vi "LV_MQTT_MDML_example.vi"() -> ()   [LabVIEW 2018]
uses:
  Downloads/mqtt_lv2013_201708181938/mqtt_lv2013/mqtt Folder/src/class/mqtt/mqttTypedef/mqttConnectionStatus.ctl
  Downloads/mqtt_lv2013_201708181938/mqtt_lv2013/mqtt Folder/src/class/mqtt/mqttTypedef/mqttConnectionMeta.ctl
  Downloads/mqtt_lv2013_201708181938/mqtt_lv2013/mqtt Folder/src/class/mqtt/mqttTypedef/mqttQOSlevel.ctl
  Downloads/mqtt_lv2013_201708181938/mqtt_lv2013/mqtt Folder/src/class/mqtt/mqttTypedef/mqttWillInformation.ctl
  vector_data.ctl
  query_part.ctl
  Downloads/mqtt_lv2013_201708181938/mqtt_lv2013/mqtt Folder/src/class/mqtt/mqtt.lvclass
panel:
  in  "Experiment ID 3":string
  in  "connMeta 7":T1
  in  "Device ID":string="DEVICE_A"
  in  "Experiment ID 2":string
  in  "Device ID":string
  in  "connMeta 6":T1
  in  "User Info":T3={"User Name"="test", "Password"="testtest"}
  in  "client":string
  in  "connMeta 5":T1
  in  "Experiment ID3":string
  in  "Configuration Filepath":path
  in  "Experiment ID":string
  in  "Experiment ID2":string
  in  "connMeta 4":T1
  out "error out 2":errorcluster
  in  "connMeta 3":T1
  out "sessionPresent":bool
  out "connStatus":T4
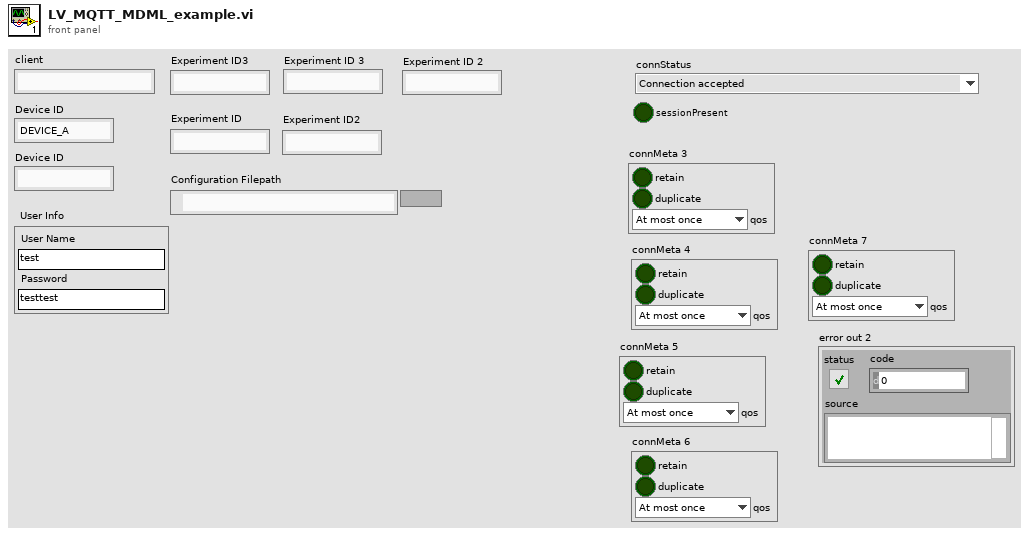
[diagram p1: front panel]
types:
  T1 = typedef "mqttConnectionMeta.ctl" = cluster{"retain":bool, "duplicate":bool, "qos":T2}
  T2 = typedef "mqttQOSlevel.ctl" = enum8{"At most once", "At least once", "Exactly once", "Reserved"}
  T3 = typedef "mqttWillInformation.ctl" = cluster{"User Name":string, "Password":string}
  T4 = typedef "mqttConnectionStatus.ctl" = enum16{"Connection accepted", "Connection refused: unacceptable protocol version", "Connection refused: identifier rejected", "Connection refused: Server unavailable", "Connection refused: bad user name or password", "Connection refused: not authorized"}
  T5 = typedef "query_part.ctl" = cluster{"device":string, "last":dbl, "variables":string[]}
  T6 = typedef "vector_data.ctl" = cluster{"wavelength":dbl[], "intensity":dbl[]}
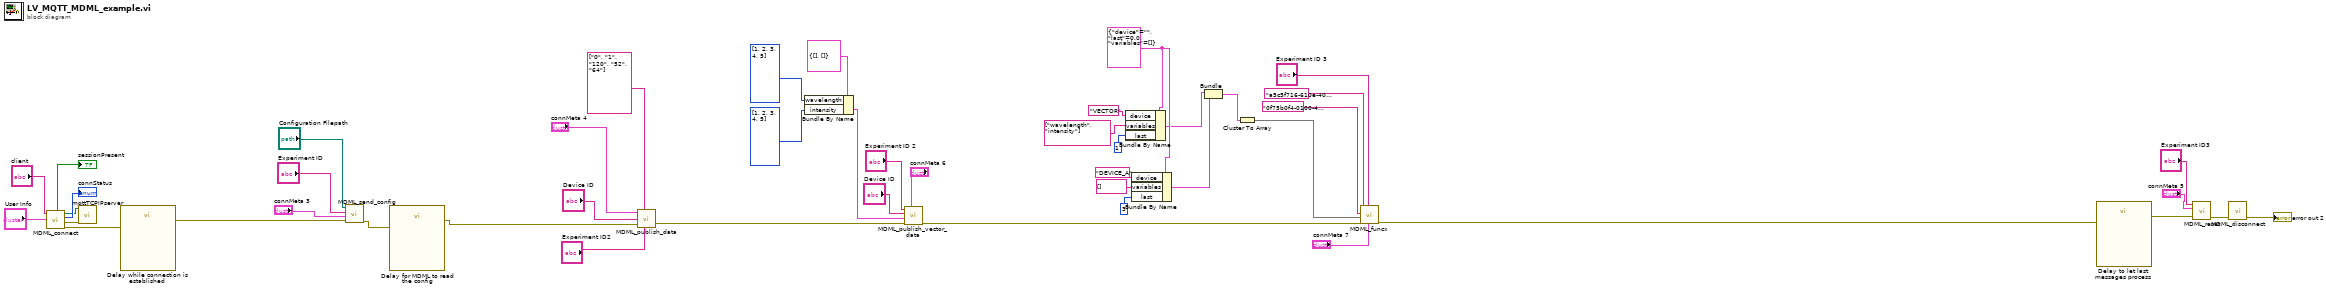
[diagram p0: block diagram]
diagram:
  w5 = T5 {"device"="", "last"=0.0, "variables"=[]} ("input cluster")
  n1 = call "MDML_connect.vi"("User Info"="User Info", "client"="client") -> ("error out"=w26:errorcluster, "error out 2"=w27:errorcluster, "connStatus"=→"connStatus":T4, "mqtt out"=w28:refnum<class "mqtt.lvclass">, "sessionPresent"=→"sessionPresent":bool)  [unwired: 5 in]
  n2 = call "mqttTCPIPserver.vi"("mqtt.lvclass"=w28, "error in (no error)"=w27) -> ()  [unwired: 12 in, 2 out]
  n3 = call "Delay while connection is established"("error in (no error)"=w26) -> ("error out"=w30:errorcluster)  [unwired: 10 in]
  n4 = call "MDML_send_config.vi"("error in (no error)"=w30, "connMeta 3"="connMeta 3", "Experiment ID"="Experiment ID", "Configuration filepath"="Configuration Filepath") -> ("error out"=w31:errorcluster)  [unwired: 7 in]
  n5 = call "Delay for MDML to read the config"("error in (no error)"=w31) -> ("error out"=w45:errorcluster)  [unwired: 10 in]
  n6 = call "MDML_publish_data.vi"("connMeta 4"="connMeta 4", "Data"=string[] ["0", "1", "120", "52", "64"] ("array"), "Device ID"="Device ID", "error in (no error)"=w45, "Experiment ID"="Experiment ID2") -> ("error out"=w20:errorcluster)  [unwired: 1 in]
  n7 = Bundle By Name(cluster=T6 {"wavelength"=[], "intensity"=[]}, "wavelength"=i32[] [1, 2, 3, 4, 5], "intensity"=i32[] [1, 2, 3, 4, 5]) -> (w21:T6)
  n8 = call "MDML_publish_vector_data.vi"("connMeta 6"="connMeta 6", "error in (no error)"=w20, "data"=w21, "Device ID"="Device ID", "Experiment ID in"="Experiment ID 2") -> ("error out"=w17:errorcluster)  [unwired: 6 in]
  n9 = Bundle By Name(cluster=w5, "device"="VECTOR", "variables"=string[] ["wavelength", "intensity"], "last"=1) -> (w4:T5)
  n10 = Bundle By Name(cluster=w5, "device"="DEVICE_A", "variables"=string[] [], "last"=3) -> (w3:T5)
  n11 = Bundle("input cluster"=w4, "input cluster"=w3) -> (w2:cluster{"input cluster":T5, "input cluster":T5})  [unwired: 1 in]
  n12 = Cluster To Array(cluster=w2) -> (array=w1:T5[])
  n13 = call "MDML_funcx.vi"("connMeta 7"="connMeta 7", "Experiment ID 3"="Experiment ID 3", "error in (no error)"=w17, "queries"=w1, "String 2"="0f75b0f4-0100-44eb-a689-e0abdc14a0e5", "String"="a5c5f716-610e-40e1-9b9c-05c4b9a0a102") -> ("error out"=w16:errorcluster)  [unwired: 5 in]
  n14 = call "Delay to let last messages process"("error in (no error)"=w16) -> ("error out"=w32:errorcluster)  [unwired: 10 in]
  n15 = call "MDML_reset.vi"("error in (no error)"=w32, "connMeta 5"="connMeta 5", "Experiment ID3"="Experiment ID3") -> ("error out"=w35:errorcluster)  [unwired: 8 in]
  n16 = call "MDML_disconnect.vi"("error in (no error)"=w35) -> ("error out"=→"error out 2":errorcluster)  [unwired: 10 in]
